vi "Build FIFO SPI Message.vi"(8 "SPI Command":T2, 9 "Chip Select":u8, 10 "Slot #":T1 max=15, 11 "Rack #":u8) -> (3 "FIFO SPI Message":u64 format="%b")   [LabVIEW 2014, in "SLSC configuration Shared.lvlib"]
uses:
  SLSC configuration Shared.lvlib
  MCP23S17/SPI Command.ctl
  Slot #.ctl
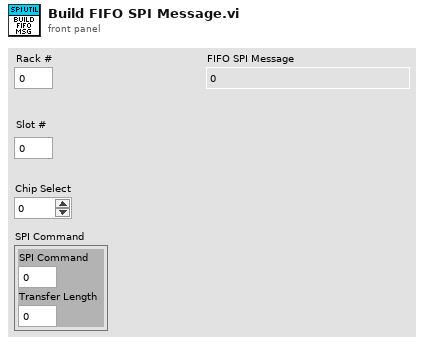
[diagram p1: front panel]
types:
  T1 = typedef "SLSC configuration Shared.lvlib/Slot #.ctl" = u8
  T2 = typedef "SLSC configuration Shared.lvlib/SPI Command.ctl" = cluster{"SPI Command":u32, "Transfer Length":u8}
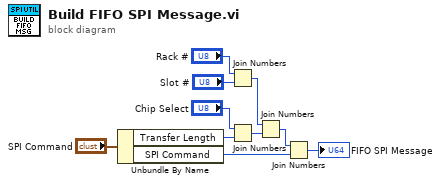
[diagram p0: block diagram]
diagram:
  n1 = Unbundle By Name("SPI Command") -> ("Transfer Length"=w4:u8, "SPI Command"=w5:u32)
  n2 = Join Numbers(hi="Rack #", lo="Slot #") -> ((hi.lo)=w1:u16)
  n3 = Join Numbers(hi="Chip Select", lo=w4) -> ((hi.lo)=w3:u16)
  n4 = Join Numbers(hi=w1, lo=w3) -> ((hi.lo)=w2:u32)
  n5 = Join Numbers(hi=w2, lo=w5) -> ((hi.lo)=→"FIFO SPI Message":u64)
